vi "绘制正方形.vi"(8 "error in (no error)":errorcluster caption="错误输入（无错误）", 11 "判定范围":string[][](table)) -> (0 "error out":errorcluster caption="错误输出", 3 "判定框":cluster{"横坐标":dbl[], "纵坐标":dbl[]}[](array[cluster]))   [LabVIEW 2018]
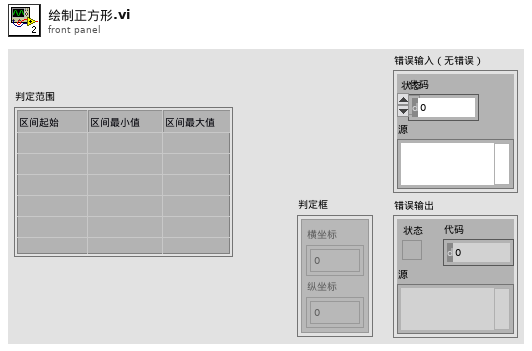
[diagram p1: front panel]
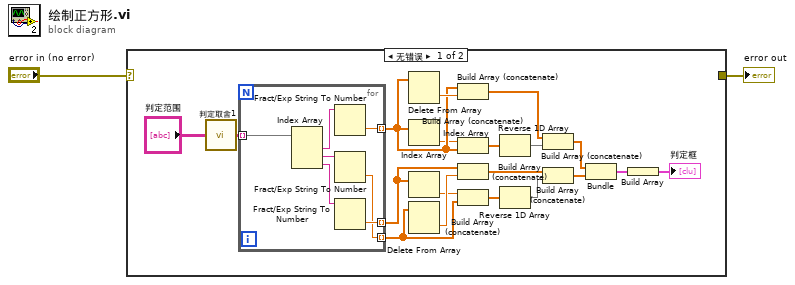
[diagram p0: block diagram]
diagram:
  n1 = case shown="无错误" "error in (no error)" {
    selector: "error in (no error)" -> [_ w29]
    tunnel: [_ w29] -> w1
    frame No Error {
      n2 = call "判定取舍1.vi"("输入表格"="判定范围") -> ("输出表格"=w21:string[][])
      n3 = for {
        tunnel: w21 -> [w28] mode=indexing
        tunnel: [w26] -> w17 mode=indexing
        tunnel: [w23] -> w18 mode=indexing
        tunnel: [w22] -> w15 mode=indexing
        n4 = Index Array(array=w28) -> (element #1=w27:string, element #2=w25:string, element #3=w24:string)  [unwired: 3 in]
        n5 = Fract/Exp String To Number(string=w27) -> (number=w26:dbl)  [unwired: 3 in, 1 out]
        n6 = Fract/Exp String To Number(string=w25) -> (number=w22:dbl)  [unwired: 3 in, 1 out]
        n7 = Fract/Exp String To Number(string=w24) -> (number=w23:dbl)  [unwired: 3 in, 1 out]
      }
      n8 = Delete From Array(array=w17) -> (deleted portion=w20:dbl)  [unwired: 2 in, 1 out]
      n9 = Index Array(array=w17) -> (element=w16:dbl)  [unwired: 1 in]
      n10 = Index Array(array=w18) -> (element=w14:dbl)  [unwired: 1 in]
      n11 = Delete From Array(array=w15) -> (deleted portion=w19:dbl)  [unwired: 2 in, 1 out]
      n12 = Build Array (concatenate)(w17, w20) -> (w11:dbl[])
      n13 = Build Array (concatenate)(w16, w17) -> (w10:dbl[])
      n14 = Build Array (concatenate)(w18, w19) -> (w9:dbl[])
      n15 = Build Array (concatenate)(w14, w15) -> (w8:dbl[])
      n16 = Reverse 1D Array(array=w10) -> (reversed array=w6:dbl[])
      n17 = Reverse 1D Array(array=w8) -> (reversed array=w7:dbl[])
      n18 = Build Array (concatenate)(w11, w6) -> (w5:dbl[])
      n19 = Build Array (concatenate)(w9, w7) -> (w4:dbl[])
      n20 = Bundle(w5, w4) -> (w3:cluster{dbl[], dbl[]})  [unwired: 1 in]
      n21 = Build Array(w3) -> (→"判定框":cluster{dbl[], dbl[]}[])
    }
    frame Error {
    }
  }
  "error out" <- w1
